vi "Drive Command Handler Temp.vi"(10 "Array":bool[](array[boolean]), 11 "Axes":dbl[](array[numeric])) -> ()   [LabVIEW 2019]
uses:
  Implementation/Drive Base Operations.ctl
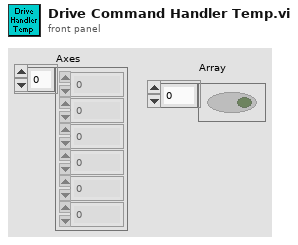
[diagram p1: front panel]
types:
  T1 = typedef "Drive Base Operations.ctl" = enum16{"Reserve", "Read Current", "Immediate", "Limelight"}
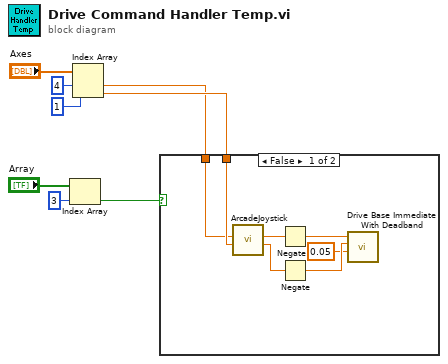
[diagram p0: block diagram]
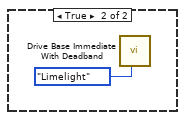
[diagram p2: hidden frame]
diagram:
  n1 = Index Array(array="Array", index=3) -> (element=w3:bool)
  n2 = Index Array(array="Axes", index #1=4 ("index"), index #2=1 ("index")) -> (element #1=w1:dbl, element #2=w2:dbl)
  n3 = case shown="False" w3 {
    tunnel: w2 -> [w10 _]
    tunnel: w1 -> [w9 _]
    frame False {
      n4 = call "ArcadeJoystick.vi"("Y axis value"=w10, "X axis value"=w9) -> ("Right Motor Value"=w13:dbl, "Left Motor Value"=w12:dbl)  [unwired: 8 in]
      n5 = Negate(x=w12) -> (-x=w14:dbl)
      n6 = Negate(x=w13) -> (-x=w15:dbl)
      n7 = call "Drive Base Immediate With Deadband.vi"("Deadband Value"=0.05, "Right Setpoint"=w15, "Left Setpoint"=w14) -> ()  [unwired: 8 in, 1 out]
    }
    frame True {
      n8 = call "Drive Base Immediate With Deadband.vi"("Operation"=Drive_Base_Operations."Limelight") -> ()  [unwired: 10 in, 1 out]
    }
  }
